vi "Global 1.vi"() -> ()   [LabVIEW 2014]
panel:
  in  "yCol":i32
  in  "xCol":i32
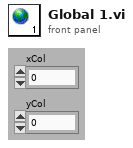
[diagram p1: front panel]
diagram:
